vi "Int32Array Destroy.vi"(8 "error in (no error)":errorcluster, 11 "Int32Array DVR in":refnum<data-value>) -> (0 "error out":errorcluster)   [LabVIEW 2010, in "MDSplus.lvlib"]
uses:
  <vilib>/MDSplus/Library/MDSplus.lvlib
  <vilib>/MDSplus/Classes/Data_Class/Array_Class/Int32Array_Class/Int32Array.lvclass
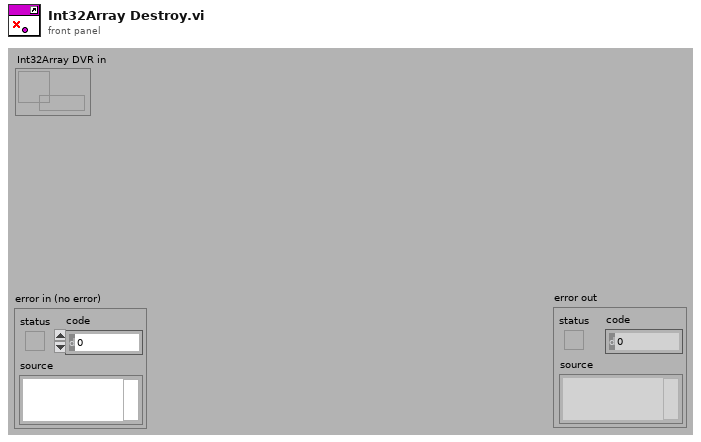
[diagram p1: front panel]
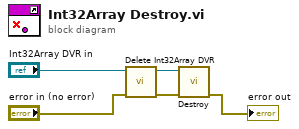
[diagram p0: block diagram]
diagram:
  n1 = call <vilib>:"Delete Int32Array DVR.vi"("error in (no error)"="error in (no error)", "Int32Array DVR in"="Int32Array DVR in") -> ("error out"=w2:errorcluster, "Int32Array out"=w3:refnum<class "Int32Array.lvclass">)  [unwired: 8 in]
  n2 = call-dynamic "Destroy.vi"("error in (no error)"=w2, "Int32Array in"=w3) -> ("error out"=→"error out":errorcluster)  [unwired: 9 in]
